vi "Backsave Individual Items.vi"(8 "Error In":errorcluster, 11 "Revert Config":T1={"Revert Paths"={"Archive Path"=path "D:/workspace/revert/todo/todo.zip", "Unzip Directory"=path "D:/workspace/revert/unzip", "Backsave Directory"=path "D:/workspace/revert/backsave", "Output Archive"=path "D:/workspace/revert/output/out.zip", "Backsave Common Directory"=path "D:/workspace/revert/backsave"}, "LabVIEW Files"={"Projects"=[], "Libraries"=[], "Classes"=[], "XControls"=[], "VIs and Controls"=[], "Non LV Files"=[]}, "LabVIEW Version"=enum."8.0"}) -> (0 "Error Out":errorcluster, 2 "Warnings":string[](array[string]), 3 "Revert Config":T1={"Revert Paths"={"Archive Path"=path "D:/workspace/revert/todo/todo.zip", "Unzip Directory"=path "D:/workspace/revert/unzip", "Backsave Directory"=path "D:/workspace/revert/backsave", "Output Archive"=path "D:/workspace/revert/output/out.zip", "Backsave Common Directory"=path "D:/workspace/revert/backsave"}, "LabVIEW Files"={"Projects"=[], "Libraries"=[], "Classes"=[], "XControls"=[], "VIs and Controls"=[], "Non LV Files"=[]}, "LabVIEW Version"=enum."8.0"})   [LabVIEW 2013, in "LVH-Revert.lvlib"]
uses:
  <vilib>/LabVIEW Hacker/Revert/LVH-Revert.lvlib
  <vilib>/LabVIEW Hacker/Revert/Type Defs/Revert Config.ctl
  <vilib>/LabVIEW Hacker/Revert/Type Defs/Paths.ctl
  <vilib>/LabVIEW Hacker/Revert/Type Defs/LabVIEW Files.ctl
  <vilib>/LabVIEW Hacker/LVH-Toolbox/Common/Private/Type Defs/LabVIEW Version.ctl
  <vilib>/LabVIEW Hacker/LVH-Toolbox/Common/LVH-Common.lvlib
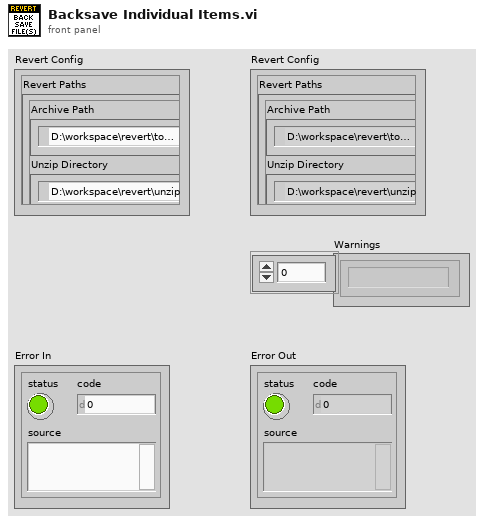
[diagram p1: front panel]
types:
  T1 = typedef "LVH-Revert.lvlib/Revert Config.ctl" = cluster{"Revert Paths":T2, "LabVIEW Files":T3, "LabVIEW Version":T4}
  T2 = typedef "LVH-Revert.lvlib/Paths.ctl" = cluster{"Archive Path":path, "Unzip Directory":path, "Backsave Directory":path, "Output Archive":path, "Backsave Common Directory":path}
  T3 = typedef "LVH-Revert.lvlib/LabVIEW Files.ctl" = cluster{"Projects":path[], "Libraries":path[], "Classes":path[], "XControls":path[], "VIs and Controls":path[], "Non LV Files":path[]}
  T4 = typedef "LVH-Toolbox.lvlib/LVH-Common.lvlib/LabVIEW Version.ctl" = enum16{"8.0", "8.2", "8.6", "9.0", "10.0", "11.0", "12.0", "13.0"}
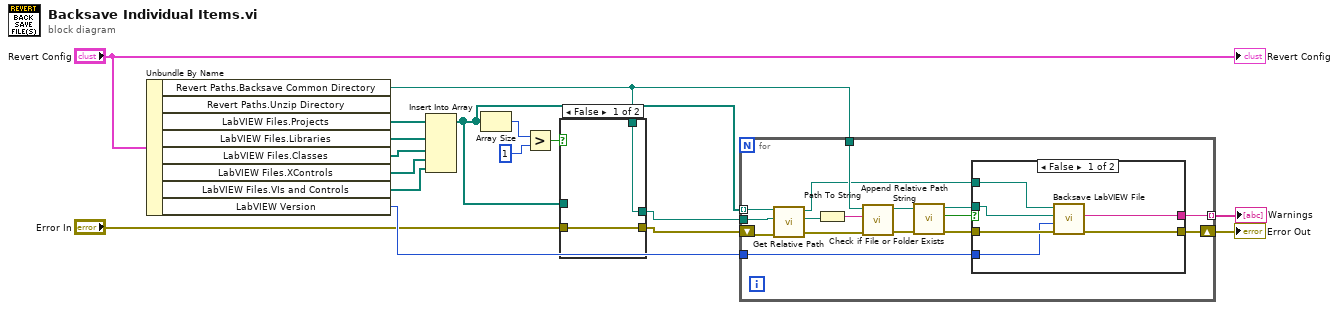
[diagram p0: block diagram]
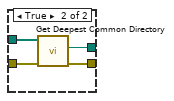
[diagram p2: hidden frame]
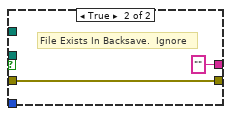
[diagram p3: hidden frame]
diagram:
  n1 = Unbundle By Name("Revert Config") -> ("Revert Paths.Backsave Common Directory"=w1:path, "LabVIEW Files.Projects"=w17:path[], "LabVIEW Files.Libraries"=w16:path[], "LabVIEW Files.Classes"=w15:path[], "LabVIEW Files.XControls"=w14:path[], "LabVIEW Files.VIs and Controls"=w13:path[], "LabVIEW Version"=w12:T4)  [unwired: 1 out]
  n2 = Insert Into Array(array=w17, new element #1=w16, new element #2=w15, new element #3=w14, new element #4=w13) -> (w2:path[])  [unwired: 1 in]
  n3 = Array Size(array=w2) -> (size(s)=w8:i32)
  n4 = Greater?(x=w8, y=1) -> (0:w6:bool)
  n5 = case shown="False" w6 {
    tunnel: [w19 w23] -> w4
    tunnel: [w18 w22] -> w3
    tunnel: "Error In" -> [w19 w21]
    tunnel: w2 -> [_ w20]
    tunnel: w1 -> [w18 _]
    frame False {
    }
    frame True {
      n6 = call <vilib>:"Get Deepest Common Directory.vi"("Error In"=w21, "File Paths"=w20) -> ("Error Out"=w23:errorcluster, "Deepest Common Path"=w22:path)  [unwired: 7 in, 1 out]
    }
  }
  n7 = for {
    tunnel: w2 -> [w39] mode=indexing
    tunnel: w1 -> [w34]
    tunnel: w12 -> [w26]
    shift-right: [w27] -> w10
    shift-left: w4 -> [w38]
    tunnel: [w25] -> w9 mode=indexing
    tunnel: w3 -> [w24]
    n8 = call <vilib>:"Get Relative Path.vi"("Error In"=w38, "Relative Path Root"=w24, "File / Folder"=w39) -> ("Error Out"=w35:errorcluster, "Relative Path"=w37:path, "Duplicate File / Folder"=w29:path)  [unwired: 6 in]
    n9 = Path To String(path=w37) -> (string=w36:string)
    n10 = call <vilib>:"Append Relative Path String.vi"("Error In"=w35, "Relative Path"=w36, "Base Path"=w34) -> ("Error Out"=w32:errorcluster, "Absolute Path"=w33:path)  [unwired: 7 in]
    n11 = call <vilib>:"Check if File or Folder Exists.vi"("error in (no error)"=w32, "path"=w33) -> ("error out"=w30:errorcluster, "file or folder exists?"=w31:bool, "dup path"=w28:path)  [unwired: 7 in]
    n12 = case shown="False" w31 {
      tunnel: w30 -> [w45 w47]
      tunnel: w29 -> [w44 _]
      tunnel: w28 -> [w43 _]
      tunnel: [w42 w47] -> w27
      tunnel: w26 -> [w41 _]
      tunnel: [w40 "" ("Warnings")] -> w25
      frame False {
        n13 = call <vilib>:"Backsave LabVIEW File.vi"("Error In"=w45, "LabVIEW Version"=w41, "Destination Path"=w43, "LabVIEW File"=w44) -> ("Error Out"=w42:errorcluster, "Warnings"=w40:string)  [unwired: 6 in]
      }
      frame True {
        # "File Exists In Backsave.  Ignore"
      }
    }
  }
  "Error Out" <- w10
  "Warnings" <- w9
  "Revert Config" <- "Revert Config"
